vi "BKP-891 LCR Meter_Create.vi"(0 "reference in":refnum<class "BKP-891 LCR Meter.lvclass">, 2 "VISA resource name":refnum<visa-resource-name>, 3 "Serial Configuration":cluster{"Baud Rate":u32}={"Baud Rate"=57600} {"Baud Rate" items=["4800"=4800, "9600"=9600, "19200"=19200, "38400"=38400, "57600"=57600]}, 5 "error in (no error)":errorcluster) -> (13 "ProcessViRef":refnum<vi>, 14 "reference out":refnum<class "BKP-891 LCR Meter.lvclass">, 19 "error out":errorcluster)   [LabVIEW 2018, in "BKP-891 LCR Meter.lvclass"]
uses:
  BKP-891 LCR Meter.lvclass
  controls/IO Signal List.ctl
  <instrlib>/BK Precision 891/BK Precision 891.lvlib
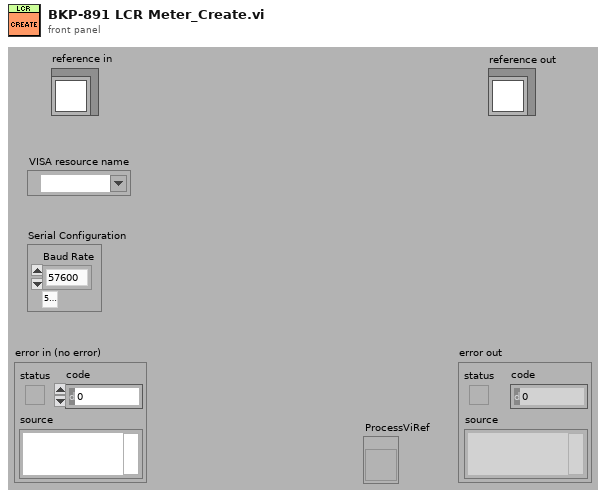
[diagram p1: front panel]
types:
  T1 = typedef "IO Signal List.ctl" = enum16{"Timestamp", "PSU_FB_U_VDC", "PSU_FB_I_AMP", "PSU_FB_W_WATT", "PSU_CMD_U_VDC", "PSU_CMD_I_AMP", "PSU_CMD_OUTPUT", "LCR_PRIMARY", "LCR_SECONDARY", "UV_R_mOhm", "UW_R_mOhm", "VW_R_mOhm", "UV_L_µH", "UW_L_µH", "VW_L_µH", "U_U_VDC", "V_U_VDC", "W_U_VDC", "U_I_AMP", "V_I_AMP", "W_I_AMP", "PWM_CMD_DC_%", "PWM_CMD_VDC", "PWM_CMD_Hz", "PWM_FB_DC_%", "PWM_FB_VDC", "PWM_FB_Hz", "DO_RELAY_U_LCR_A", "DO_RELAY_V_LCR_A", "DO_RELAY_V_LCR_B", "DO_RELAY_W_LCR_B", "DIFF_UV_UW_L_µH", "DIFF_UV_VW_L_µH", "DIFF_UW_VW_L_µH", "DIFF_UV_UW_R_mOhm", "DIFF_UV_VW_R_mOhm", "DIFF_UW_VW_R_mOhm", "DIFF_UV_U_VDC", "DIFF_UW_U_VDC", "DIFF_VW_U_VDC"}
  T2 = typedef "BKP-891 LCR Meter.lvclass/ObjectAttributes.ctl" = cluster{"VISA resource name":refnum<visa-resource-name>, "Simulated?":bool, "Latest Values":dbl[], "Signal List":T1[], "Tare Offset":dbl[], "Range":u16, "Measurement Speed":u16, "Function":u16, "Signal Frequency (Hz)":dbl, "Signal Level (Vrms)":u8, "UVW Mode":enum16{"None", "UV", "UW", "VW"}, "LR Mode":T3, "Primary Parameter":string, "Secondary Parameter":string}
  T3 = typedef "LR Mode.ctl" = enum16{"R - Resistance", "L - Inductance"}
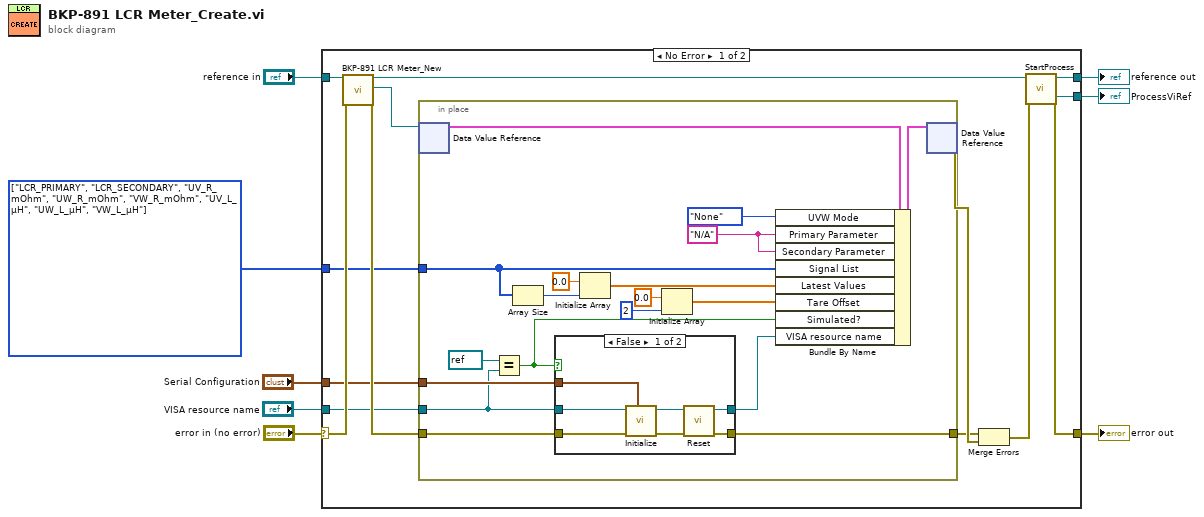
[diagram p0: block diagram]
diagram:
  w2 = T1[] [enum."LCR_PRIMARY", enum."LCR_SECONDARY", enum."UV_R_mOhm", enum."UW_R_mOhm", enum."VW_R_mOhm", enum."UV_L_µH", enum."UW_L_µH", enum."VW_L_µH"] items=["Timestamp", "PSU_FB_U_VDC", "PSU_FB_I_AMP", "PSU_FB_W_WATT", "PSU_CMD_U_VDC", "PSU_CMD_I_AMP", "PSU_CMD_OUTPUT", "LCR_PRIMARY", "LCR_SECONDARY", "UV_R_mOhm", "UW_R_mOhm", "VW_R_mOhm", "UV_L_µH", "UW_L_µH", "VW_L_µH", "U_U_VDC", "V_U_VDC", "W_U_VDC", "U_I_AMP", "V_I_AMP", "W_I_AMP", "PWM_CMD_DC_%", "PWM_CMD_VDC", "PWM_CMD_Hz", "PWM_FB_DC_%", "PWM_FB_VDC", "PWM_FB_Hz", "DO_RELAY_U_LCR_A", "DO_RELAY_V_LCR_A", "DO_RELAY_V_LCR_B", "DO_RELAY_W_LCR_B", "DIFF_UV_UW_L_µH", "DIFF_UV_VW_L_µH", "DIFF_UW_VW_L_µH", "DIFF_UV_UW_R_mOhm", "DIFF_UV_VW_R_mOhm", "DIFF_UW_VW_R_mOhm", "DIFF_UV_U_VDC", "DIFF_UW_U_VDC", "DIFF_VW_U_VDC"] ("Signal List")
  n1 = case shown="No Error" "error in (no error)" {
    selector: "error in (no error)" -> [w21 w51]
    tunnel: [w13 w51] -> w7
    tunnel: "reference in" -> [w22 w50]
    tunnel: [w15 w50] -> w5
    tunnel: "VISA resource name" -> [w12 _]
    tunnel: [w11 _] -> w3
    tunnel: w2 -> [w10 _]
    tunnel: "Serial Configuration" -> [w9 _]
    frame No Error {
      n2 = call "BKP-891 LCR Meter_New.vi"("reference in"=w22, "error in (no error)"=w21) -> ("reference out"=w16:refnum<class "BKP-891 LCR Meter.lvclass">, "DVRRefOut"=w19:refnum<data-value>, "error out"=w18:errorcluster)  [unwired: 14 in, 1 out]
      n3 = in-place {
        in-place-border: w18 -> [w38]
        in-place-border: [w37] -> w17
        in-place-border: w12 -> [w33]
        in-place-border: w10 -> [w27]
        in-place-border: w9 -> [w34]
        w29 = "N/A" ("Primary Parameter")
        n4 = in-place-dvr #1(w19) -> (w39:T2)  [unwired: 1 out]
        n5 = Equal?(x=refnum<visa-resource-name> refnum, y=w33) -> (x = y?=w30:bool)
        n6 = Array Size(array=w27) -> (size(s)=w26:i32)
        n7 = case shown="False" w30 {
          tunnel: w38 -> [w47 w48]
          tunnel: w33 -> [w46 w49]
          tunnel: [w43 w49] -> w31
          tunnel: [w42 w48] -> w37
          tunnel: w34 -> [w41 _]
          frame False {
            n8 = call <instrlib>:"Initialize.vi"("Serial Configuration"=w41, "error in (no error)"=w47, "VISA resource name"=w46) -> ("error out"=w45:errorcluster, "VISA resource name out"=w44:refnum<visa-resource-name>)  [unwired: 7 in]
            n9 = call <instrlib>:"Reset.vi"("error in (no error)"=w45, "VISA resource name"=w44) -> ("error out"=w42:errorcluster, "VISA resource name out"=w43:refnum<visa-resource-name>)  [unwired: 8 in]
          }
          frame True {
          }
        }
        n10 = Initialize Array(0.0 ("element"), w26) -> (w35:dbl[])
        n11 = Initialize Array(0.0 ("element"), 2 ("dimension size")) -> (w23:dbl[])
        n12 = Bundle By Name(cluster=w39, "UVW Mode"=enum16{"None", "UV", "UW", "VW"}."None", "Primary Parameter"=w29, "Secondary Parameter"=w29, "Signal List"=w27, "Latest Values"=w35, "Tare Offset"=w23, "Simulated?"=w30, "VISA resource name"=w31) -> (w40:T2)
        n13 = in-place-dvr #1(w40) -> (w20:errorcluster)  [unwired: 1 out]
      }
      n14 = Merge Errors(w17, w20) -> (w14:errorcluster)
      n15 = call "StartProcess.vi"("reference in"=w16, "error in (no error)"=w14) -> ("reference out"=w15:refnum<class "BKP-891 LCR Meter.lvclass">, "ProcessViRef"=w11:refnum<vi>, "error out"=w13:errorcluster)  [unwired: 13 in, 2 out]
    }
    frame Error {
      # "VI-TechBaseTemplate_Simple_6x8x6"
    }
  }
  "error out" <- w7
  "reference out" <- w5
  "ProcessViRef" <- w3
